vi "SCPE.vi"(7 "FileName":string, 10 "IV array":dbl[][](array[numeric])) -> (0 "Rsh":dbl, 1 "Rs":dbl, 2 "Voc":dbl, 3 "Isc":dbl, 5 "Fill Factor":dbl, 6 "n":dbl)   [LabVIEW 2020]
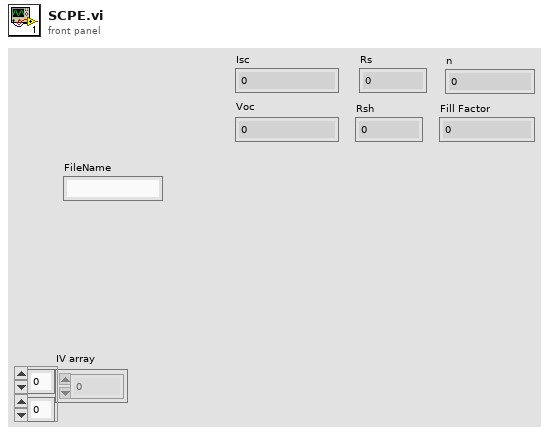
[diagram p1: front panel]
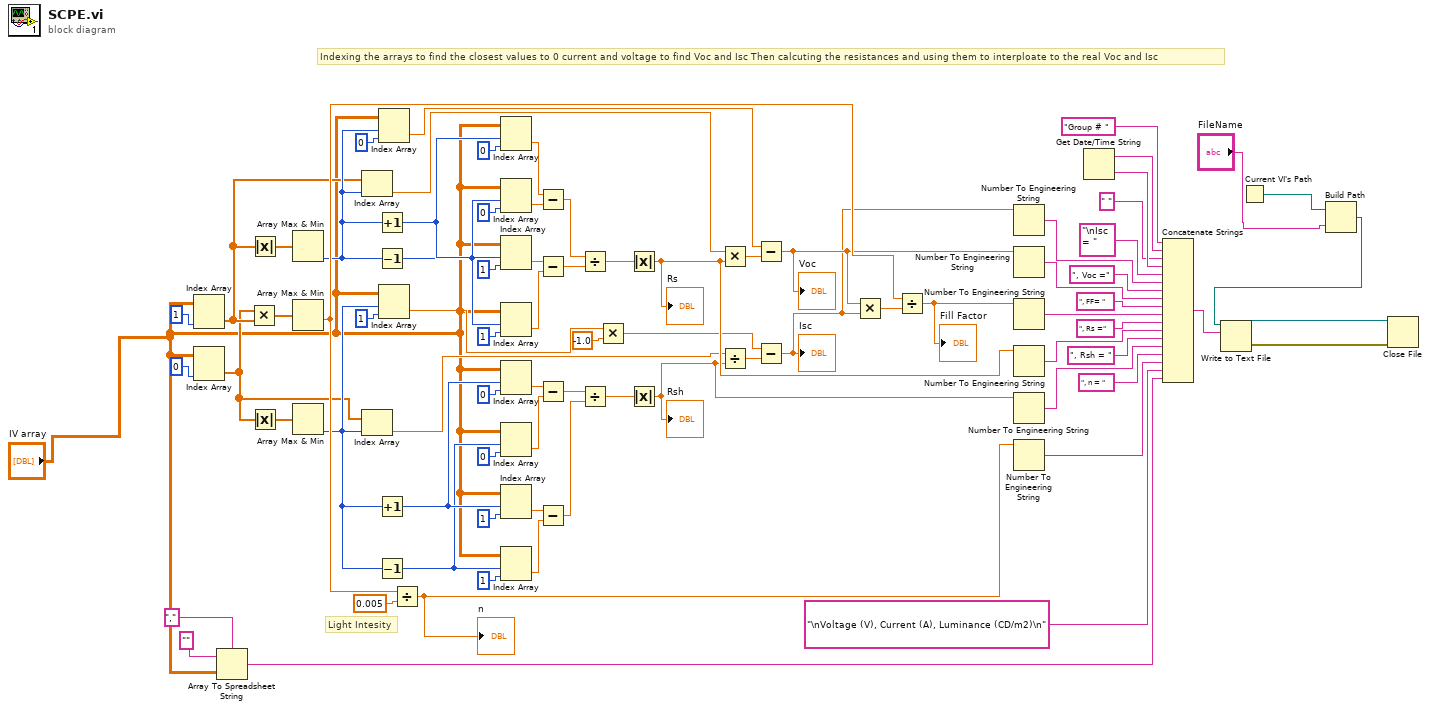
[diagram p0: block diagram]
diagram:
  # "Indexing the arrays to find the closest values to 0 current and voltage to find Voc and Isc Then calcuting the resistances and using them to interploate to the real Voc and Isc"
  # "Light Intesity"
  n1 = Index Array(array="IV array", index (col)=1 ("disabled index (col)")) -> (element=w17:dbl[])  [unwired: 1 in]
  n2 = Index Array(array="IV array", index (col)=0 ("disabled index (col)")) -> (element=w5:dbl[])  [unwired: 1 in]
  n3 = Array To Spreadsheet String(delimiter (Tab)=",", array="IV array", 3:"" ("format string")) -> (spreadsheet string=w23:string)
  n4 = Multiply(x=w5, y=w17) -> (x*y=w47:dbl[])
  n5 = Absolute Value(x=w17) -> (abs(x)=w75:dbl[])
  n6 = Absolute Value(x=w5) -> (abs(x)=w80:dbl[])
  n7 = Array Max & Min(array=w75) -> (min index (indices)=w18:i32)  [unwired: 3 out]
  n8 = Array Max & Min(array=w47) -> (min value=w44:dbl)  [unwired: 3 out]
  n9 = Array Max & Min(array=w80) -> (min index (indices)=w6:i32)  [unwired: 3 out]
  n10 = Index Array(array=w17, index=w18) -> (element=w16:dbl)
  n11 = Index Array(array=w5, index=w6) -> (element=w7:dbl)
  n12 = Increment(x=w18) -> (x+1=w60:i32)
  n13 = Decrement(x=w18) -> (x-1=w55:i32)
  n14 = Increment(x=w6) -> (x+1=w73:i32)
  n15 = Decrement(x=w6) -> (x-1=w68:i32)
  n16 = Index Array(array="IV array", index (row)=w18, index (col)=0 ("disabled index (col)")) -> (element=w15:dbl)
  n17 = Index Array(array="IV array", index (row)=w6, index (col)=1 ("disabled index (col)")) -> (element=w78:dbl)
  n18 = Divide(x=w44, y=0.005) -> (x/y=w25:dbl)
  "n" <- w25
  n19 = Index Array(array="IV array", index (row)=w60, index (col)=0 ("disabled index (col)")) -> (element=w54:dbl)
  n20 = Index Array(array="IV array", index (row)=w55, index (col)=0 ("disabled index (col)")) -> (element=w53:dbl)
  n21 = Index Array(array="IV array", index (row)=w60, index (col)=1 ("disabled index (col)")) -> (element=w52:dbl)
  n22 = Index Array(array="IV array", index (row)=w55, index (col)=1 ("disabled index (col)")) -> (element=w51:dbl)
  n23 = Index Array(array="IV array", index (row)=w73, index (col)=0 ("disabled index (col)")) -> (element=w67:dbl)
  n24 = Index Array(array="IV array", index (row)=w68, index (col)=0 ("disabled index (col)")) -> (element=w66:dbl)
  n25 = Index Array(array="IV array", index (row)=w73, index (col)=1 ("disabled index (col)")) -> (element=w65:dbl)
  n26 = Index Array(array="IV array", index (row)=w68, index (col)=1 ("disabled index (col)")) -> (element=w64:dbl)
  n27 = Subtract(x=w54, y=w53) -> (x-y=w50:dbl)
  n28 = Subtract(x=w52, y=w51) -> (x-y=w49:dbl)
  n29 = Subtract(x=w67, y=w66) -> (x-y=w63:dbl)
  n30 = Subtract(x=w65, y=w64) -> (x-y=w62:dbl)
  n31 = Divide(x=w50, y=w49) -> (x/y=w48:dbl)
  n32 = Divide(x=w63, y=w62) -> (x/y=w61:dbl)
  n33 = Multiply(x=w78, y=-1.0) -> (x*y=w10:dbl)
  n34 = Absolute Value(x=w48) -> (abs(x)=w12:dbl)
  "Rs" <- w12
  n35 = Absolute Value(x=w61) -> (abs(x)=w11:dbl)
  "Rsh" <- w11
  n36 = Multiply(x=w16, y=w12) -> (x*y=w14:dbl)
  n37 = Divide(x=w7, y=w11) -> (x/y=w9:dbl)
  n38 = Subtract(x=w15, y=w14) -> (x-y=w13:dbl)
  "Voc" <- w13
  n39 = Subtract(x=w10, y=w9) -> (x-y=w8:dbl)
  "Isc" <- w8
  n40 = Multiply(x=w13, y=w8) -> (x*y=w46:dbl)
  n41 = Divide(x=w44, y=w46) -> (x/y=w29:dbl)
  "Fill Factor" <- w29
  n42 = Number To Engineering String(4:w8) -> (0:w39:string)  [unwired: 3 in]
  n43 = Number To Engineering String(4:w13) -> (0:w37:string)  [unwired: 3 in]
  n44 = Number To Engineering String(4:w29) -> (0:w35:string)  [unwired: 3 in]
  n45 = Number To Engineering String(4:w12) -> (0:w33:string)  [unwired: 3 in]
  n46 = Number To Engineering String(4:w11) -> (0:w31:string)  [unwired: 3 in]
  n47 = Number To Engineering String(4:w25) -> (0:w24:string)  [unwired: 3 in]
  n48 = Get Date/Time String() -> (date string=w20:string, time string=w41:string)  [unwired: 3 in]
  n49 = Concatenate Strings("Group # ", w20, " " ("string"), w41, "\nIsc = " ("string"), w39, ", Voc =" ("string"), w37, ", FF= " ("string"), w35, ", Rs =" ("string"), w33, ", Rsh = " ("string"), w31, ", n = " ("string"), w24, "\nVoltage (V), Current (A), Luminance (CD/m2)\n" ("string"), w23) -> (w28:string)
  n50 = Current VI's Path() -> (path=w3:path)
  n51 = Build Path(base path=w3, name or relative path="FileName") -> (appended path=w2:path)
  n52 = Write to Text File(file (use dialog)=w2, text=w28) -> (refnum out=w42:refnum<file>, error out=w43:errorcluster)  [unwired: 2 in, 1 out]
  n53 = Close File(refnum=w42, error in=w43) -> ()  [unwired: 2 out]
